vi "Defaults.vi"(8 "error in (no error)":errorcluster, 11 "MB Slave in":refnum<class "iC7-INU.lvclass">) -> (0 "error out":errorcluster, 3 "MB Slave out":refnum<class "iC7-INU.lvclass">)   [LabVIEW 2021, in "iC7-INU.lvclass"]
uses:
  iC7-INU.lvclass
  C:/Program Files (x86)/National Instruments/LabVIEW 2021/user.lib/S2 Labs/Module Framework/Modules/Modbus/Modbus Slave Base/Modbus Slave Base.lvclass
  <userlib>/S2 Labs/Modbus Toolkit/TypeDefs/MB Element.ctl
  <userlib>/S2 Labs/Modbus Toolkit/TypeDefs/Endianness Type.ctl
  <userlib>/S2 Labs/Modbus Toolkit/TypeDefs/Access Type.ctl
  <userlib>/S2 Labs/Module Framework/Modules/Modbus/Modbus Slave Base/Modbus Slave Base.lvclass/Modbus Slave Base.ctl
  <userlib>/S2 Labs/Module Framework/Modules/Modbus/Modbus Slave Base/Write MB Map.vi
  MB Slave Simulator Base/MB Slave Simulator Base.lvclass
  iC7-INU.lvclass/iC7-INU.ctl
  <userlib>/S2 Labs/Modbus Toolkit/S2L Modbus API.lvclass
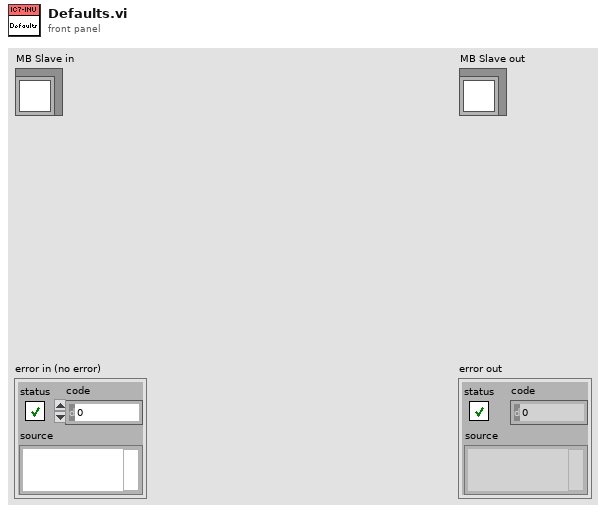
[diagram p1: front panel]
types:
  T1 = typedef "S2L Modbus API.lvclass/MB Element.ctl" = cluster{"Label":string, "Prefix":u8, "Address":u16, "Datatype":string, "Register Count":u8, "Multiplier":dbl, "Offset":dbl, "Unit":string, "Endianness":T2, "Access":T3, "LUT":string[], "Poll Rate(ms)":u16, "Mapping":cluster{"Module":string, "Channel":string}}
  T2 = typedef "Endianness Type.ctl" = enum16{"Big-Endian", "Little-Endian", "Big-Endian Byte Swap", "Little-Endian Byte Swap"}
  T3 = typedef "S2L Modbus API.lvclass/Access Type.ctl" = enum16{"R/W", "R", "W"}
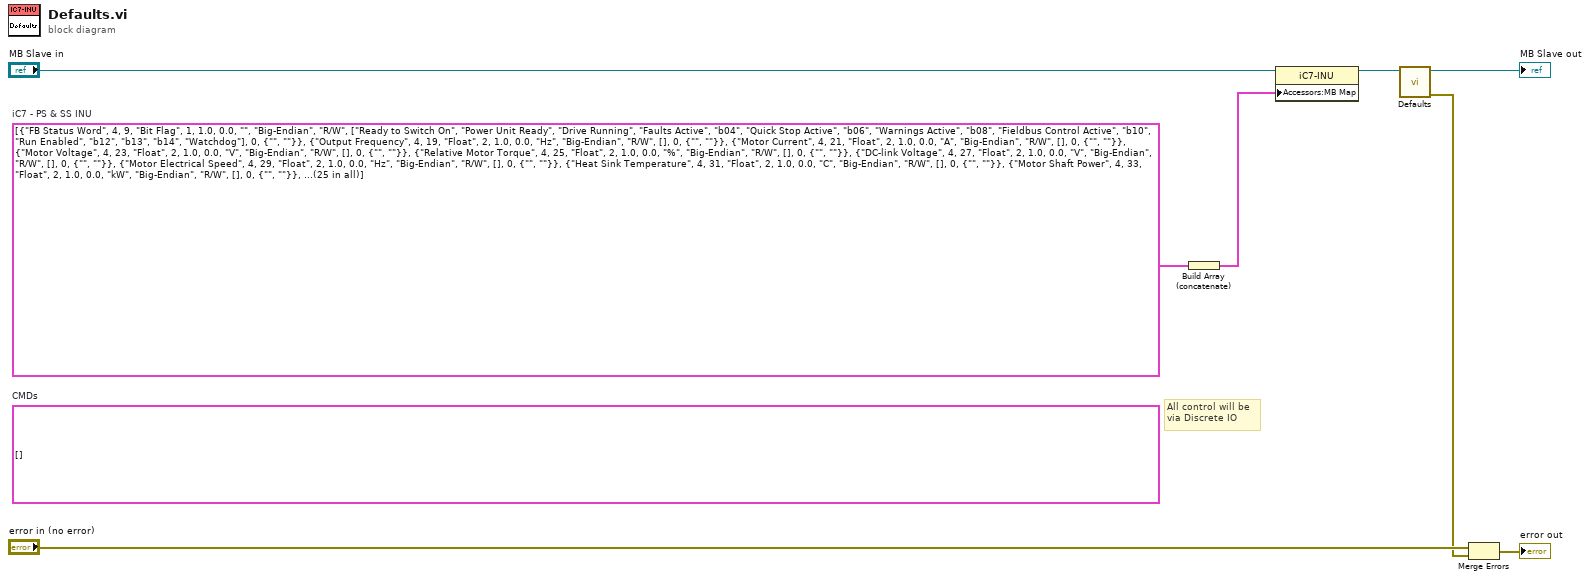
[diagram p0: block diagram]
diagram:
  (unwired) T1[] []  # CMDs
  w6 = T1[] [{"Label"="FB Status Word", "Prefix"=4, "Address"=9, "Datatype"="Bit Flag", "Register Count"=1, "Multiplier"=1.0, "Offset"=0.0, "Unit"="", "Endianness"=enum."Big-Endian", "Access"=enum."R/W", "LUT"=["Ready to Switch On", "Power Unit Ready", "Drive Running", "Faults Active", "b04", "Quick Stop Active", "b06", "Warnings Active", "b08", "Fieldbus Control Active", "b10", "Run Enabled", "b12", "b13", "b14", "Watchdog"], "Poll Rate(ms)"=0, "Mapping"={"Module"="", "Channel"=""}}, {"Label"="Output Frequency", "Prefix"=4, "Address"=19, "Datatype"="Float", "Register Count"=2, "Multiplier"=1.0, "Offset"=0.0, "Unit"="Hz", "Endianness"=enum."Big-Endian", "Access"=enum."R/W", "LUT"=[], "Poll Rate(ms)"=0, "Mapping"={"Module"="", "Channel"=""}}, {"Label"="Motor Current", "Prefix"=4, "Address"=21, "Datatype"="Float", "Register Count"=2, "Multiplier"=1.0, "Offset"=0.0, "Unit"="A", "Endianness"=enum."Big-Endian", "Access"=enum."R/W", "LUT"=[], "Poll Rate(ms)"=0, "Mapping"={"Module"="", "Channel"=""}}, {"Label"="Motor Voltage", "Prefix"=4, "Address"=23, "Datatype"="Float", "Register Count"=2, "Multiplier"=1.0, "Offset"=0.0, "Unit"="V", "Endianness"=enum."Big-Endian", "Access"=enum."R/W", "LUT"=[], "Poll Rate(ms)"=0, "Mapping"={"Module"="", "Channel"=""}}, {"Label"="Relative Motor Torque", "Prefix"=4, "Address"=25, "Datatype"="Float", "Register Count"=2, "Multiplier"=1.0, "Offset"=0.0, "Unit"="%", "Endianness"=enum."Big-Endian", "Access"=enum."R/W", "LUT"=[], "Poll Rate(ms)"=0, "Mapping"={"Module"="", "Channel"=""}}, {"Label"="DC-link Voltage", "Prefix"=4, "Address"=27, "Datatype"="Float", "Register Count"=2, "Multiplier"=1.0, "Offset"=0.0, "Unit"="V", "Endianness"=enum."Big-Endian", "Access"=enum."R/W", "LUT"=[], "Poll Rate(ms)"=0, "Mapping"={"Module"="", "Channel"=""}}, {"Label"="Motor Electrical Speed", "Prefix"=4, "Address"=29, "Datatype"="Float", "Register Count"=2, "Multiplier"=1.0, "Offset"=0.0, "Unit"="Hz", "Endianness"=enum."Big-Endian", "Access"=enum."R/W", "LUT"=[], "Poll Rate(ms)"=0, "Mapping"={"Module"="", "Channel"=""}}, {"Label"="Heat Sink Temperature", "Prefix"=4, "Address"=31, "Datatype"="Float", "Register Count"=2, "Multiplier"=1.0, "Offset"=0.0, "Unit"="C", "Endianness"=enum."Big-Endian", "Access"=enum."R/W", "LUT"=[], "Poll Rate(ms)"=0, "Mapping"={"Module"="", "Channel"=""}}, {"Label"="Motor Shaft Power", "Prefix"=4, "Address"=33, "Datatype"="Float", "Register Count"=2, "Multiplier"=1.0, "Offset"=0.0, "Unit"="kW", "Endianness"=enum."Big-Endian", "Access"=enum."R/W", "LUT"=[], "Poll Rate(ms)"=0, "Mapping"={"Module"="", "Channel"=""}}, {"Label"="Relative Motor Shaft Power", "Prefix"=4, "Address"=35, "Datatype"="Float", "Register Count"=2, "Multiplier"=1.0, "Offset"=0.0, "Unit"="%", "Endianness"=enum."Big-Endian", "Access"=enum."R/W", "LUT"=[], "Poll Rate(ms)"=0, "Mapping"={"Module"="", "Channel"=""}}, {"Label"="Fault Status Word 1-1", "Prefix"=4, "Address"=37, "Datatype"="Bit Flag", "Register Count"=1, "Multiplier"=1.0, "Offset"=0.0, "Unit"="", "Endianness"=enum."Big-Endian", "Access"=enum."R/W", "LUT"=["Over current", "DC-Link Over voltage", "DC-Link Under voltage", "Unit over temperature", "Unit under temperature", "Control card over temp", "Input phase", "Output phase", "Earth", "Fan failure", "Fieldbus issue", "HMI control lost", "Feedback failure", "Thermistor", "Auxiliary device", "External temperature measurement"], "Poll Rate(ms)"=0, "Mapping"={"Module"="", "Channel"=""}}, {"Label"="Fault Status Word 1-2", "Prefix"=4, "Address"=38, "Datatype"="Bit Flag", "Register Count"=1, "Multiplier"=1.0, "Offset"=0.0, "Unit"="", "Endianness"=enum."Big-Endian", "Access"=enum."R/W", "LUT"=["Grid side overvoltage", "Grid side undervoltage"], "Poll Rate(ms)"=0, "Mapping"={"Module"="", "Channel"=""}}, {"Label"="Fault Status Word 2", "Prefix"=4, "Address"=39, "Datatype"="Bit Flag", "Register Count"=1, "Multiplier"=1.0, "Offset"=0.0, "Unit"="", "Endianness"=enum."Big-Endian", "Access"=enum."R/W", "LUT"=["Live Zero", "Motor Overload", "Limit Supervision", "Quick stop", "Motor over temperature", "Speed error", "External Event", "Cooling monitor", "Mechanical Brake", "Safe Torque Off", "Stall Protection", "Interlocking"], "Poll Rate(ms)"=0, "Mapping"={"Module"="", "Channel"=""}}, {"Label"="Warning Status Word 1-1", "Prefix"=4, "Address"=41, "Datatype"="Bit Flag", "Register Count"=1, "Multiplier"=1.0, "Offset"=0.0, "Unit"="", "Endianness"=enum."Big-Endian", "Access"=enum."R/W", "LUT"=["Over current", "DC-Link Over voltage", "DC-Link Under voltage", "Unit over temperature", "Unit under temperature", "Control card over temp", "Input phase", "Output phase", "Earth", "Fan failure", "Fieldbus issue", "HMI control lost", "Feedback failure", "Thermistor", "Auxiliary device", "External temperature measurement"], "Poll Rate(ms)"=0, "Mapping"={"Module"="", "Channel"=""}}, {"Label"="Warning Status Word 1-2", "Prefix"=4, "Address"=42, "Datatype"="Bit Flag", "Register Count"=1, "Multiplier"=1.0, "Offset"=0.0, "Unit"="", "Endianness"=enum."Big-Endian", "Access"=enum."R/W", "LUT"=["Grid side overvoltage", "Grid side undervoltage"], "Poll Rate(ms)"=0, "Mapping"={"Module"="", "Channel"=""}}, {"Label"="Warning Status Word 2", "Prefix"=4, "Address"=43, "Datatype"="Bit Flag", "Register Count"=1, "Multiplier"=1.0, "Offset"=0.0, "Unit"="", "Endianness"=enum."Big-Endian", "Access"=enum."R/W", "LUT"=["Live Zero", "Motor Overload", "Limit Supervision", "Quick stop", "Motor over temperature", "Speed error", "External Event", "Cooling monitor", "Mechanical Brake", "Safe Torque Off", "Stall Protection", "Interlocking"], "Poll Rate(ms)"=0, "Mapping"={"Module"="", "Channel"=""}}, {"Label"="Last Fault Number", "Prefix"=4, "Address"=45, "Datatype"="U16", "Register Count"=1, "Multiplier"=1.0, "Offset"=0.0, "Unit"="", "Endianness"=enum."Big-Endian", "Access"=enum."R/W", "LUT"=[], "Poll Rate(ms)"=0, "Mapping"={"Module"="", "Channel"=""}}, {"Label"="Motor Power Limit", "Prefix"=4, "Address"=46, "Datatype"="Float", "Register Count"=1, "Multiplier"=1.0, "Offset"=0.0, "Unit"="%", "Endianness"=enum."Big-Endian", "Access"=enum."R/W", "LUT"=[], "Poll Rate(ms)"=0, "Mapping"={"Module"="", "Channel"=""}}, {"Label"="Motor Speed Feedback", "Prefix"=4, "Address"=48, "Datatype"="Float", "Register Count"=1, "Multiplier"=1.0, "Offset"=0.0, "Unit"="rpm", "Endianness"=enum."Big-Endian", "Access"=enum."R/W", "LUT"=[], "Poll Rate(ms)"=0, "Mapping"={"Module"="", "Channel"=""}}, {"Label"="DI Bit Word", "Prefix"=4, "Address"=50, "Datatype"="Bit Flag", "Register Count"=1, "Multiplier"=1.0, "Offset"=0.0, "Unit"="", "Endianness"=enum."Big-Endian", "Access"=enum."R/W", "LUT"=["b00", "b01", "b02", "Breaker Charged", "MCB Feedback"], "Poll Rate(ms)"=0, "Mapping"={"Module"="", "Channel"=""}}, {"Label"="Winding Temp 1", "Prefix"=4, "Address"=51, "Datatype"="Float", "Register Count"=1, "Multiplier"=1.0, "Offset"=0.0, "Unit"="C", "Endianness"=enum."Big-Endian", "Access"=enum."R/W", "LUT"=[], "Poll Rate(ms)"=0, "Mapping"={"Module"="", "Channel"=""}}, {"Label"="Winding Temp 2", "Prefix"=4, "Address"=53, "Datatype"="Float", "Register Count"=1, "Multiplier"=1.0, "Offset"=0.0, "Unit"="C", "Endianness"=enum."Big-Endian", "Access"=enum."R/W", "LUT"=[], "Poll Rate(ms)"=0, "Mapping"={"Module"="", "Channel"=""}}, {"Label"="Winding Temp 3", "Prefix"=4, "Address"=55, "Datatype"="Float", "Register Count"=1, "Multiplier"=1.0, "Offset"=0.0, "Unit"="C", "Endianness"=enum."Big-Endian", "Access"=enum."R/W", "LUT"=[], "Poll Rate(ms)"=0, "Mapping"={"Module"="", "Channel"=""}}, {"Label"="D Bearing Temp", "Prefix"=4, "Address"=57, "Datatype"="Float", "Register Count"=1, "Multiplier"=1.0, "Offset"=0.0, "Unit"="C", "Endianness"=enum."Big-Endian", "Access"=enum."R/W", "LUT"=[], "Poll Rate(ms)"=0, "Mapping"={"Module"="", "Channel"=""}}, {"Label"="N Bearing Temp", "Prefix"=4, "Address"=59, "Datatype"="Float", "Register Count"=1, "Multiplier"=1.0, "Offset"=0.0, "Unit"="C", "Endianness"=enum."Big-Endian", "Access"=enum."R/W", "LUT"=[], "Poll Rate(ms)"=0, "Mapping"={"Module"="", "Channel"=""}}]  # iC7 - PS & SS INU
  # "All control will be\nvia Discrete IO"
  n1 = Build Array (concatenate)(w6) -> (w7:T1[])
  n2 = property class="iC7-INU"(reference="MB Slave in", "Accessors:MB Map"=w7) -> (reference out=w4:refnum<class "iC7-INU.lvclass">)  [unwired: 1 in, 1 out]
  n3 = call-parent "Defaults.vi"("MB Slave in"=w4) -> ("error out"=w1:errorcluster, "MB Slave out"=→"MB Slave out":refnum<class "iC7-INU.lvclass">)  [unwired: 9 in]
  n4 = Merge Errors("error in (no error)", w1) -> (→"error out":errorcluster)
